vi "SwissSPAD Live_Get FLI Data Type for HDF5.vi"(8 "error in (no error)":errorcluster) -> (0 "error out":errorcluster, 3 "Data Type":string)   [LabVIEW 2021]
uses:
  SwissSPAD Live_Settings List.ctl
  SwissSPAD Live_SSx PCB Version.ctl
  SwissSPAD Live_SS2 DAQ Parameters 3.ctl
  SwissSPAD Live_SS2 Gate Definition.ctl
  SwissSPAD Live_SS3 DAQ Parameters.ctl
  SwissSPAD Live_SS3 Gate Definition.ctl
  SS3 Gate Width Definition Mode.ctl
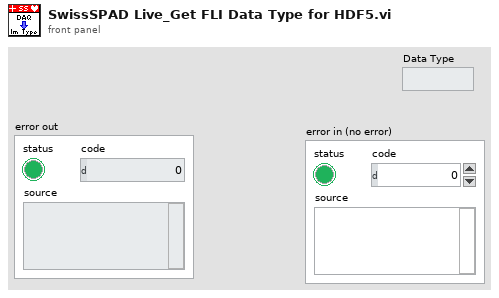
[diagram p1: front panel]
types:
  T1 = typedef "SwissSPAD Live_SSx PCB Version.ctl" = enum16{"unknown", "SS2 PCB1", "SS2 PCB2", "SS3 PCB1"}
  T2 = typedef "SwissSPAD Live_Settings List.ctl" = enum16{"FPGA:Bottom Half", "FPGA:Top Half", "FPGA:Bottom Bitfile Path", "FPGA:Top Bitfile Path", "FPGA:Bottom Bitstream Version", "FPGA:Top Bitstream Version", "FPGA:Auto Reset FPGA", "FPGA:Bottom FPGA Serial Number", "FPGA:Top FPGA Serial Number", "FPGA:Detector PCB Version", "Acquisition Parameters:Microlens", "Acquisition Parameters:SS2 DAQ Parameters", "Acquisition Parameters:Gate Configuration Array", "Acquisition Parameters:SS3 DAQ Parameters", "Acquisition Parameters:Buffer Size (# 8-bit Gates)", "File Information:File Information", "File Information:# Datasets in Series", "File Information:Scrambled File Flag", "File Information:SS3 Gate Slip Correction", "File Information:SS3 Hot Pixel Mismatch Detection", "File Information:Delay between Datasets", "File Information:Save Sum of All Gates Preview", "Image Parameters:Image ROI Information", "Image Parameters:Image Binning Options", "Image Parameters:SS3 Displayed Image", "Image Parameters:Image Display Options", "Image Parameters:Use Histogram Cursors", "Image Parameter:FPGA Data to Display", "UI Settings:Histogram Bins Number", "UI Settings:Histogram Bin Size", "UI Settings:Use Image Display Options", "UI Settings:Verbose Settings", "UI Settings:Verbose Saving"}
  T3 = typedef "SwissSPAD Live_SS2 DAQ Parameters 3.ctl" = cluster{"10 bits":bool, "# Exposure Sequences":u32, "# 1-bit Frame per Gate":u32, "Gate Shift":u32, "# Gates per Set":u32, "# Sets":u32, "Laser Period":dbl[unit], "Sync Period":dbl[unit], "Gate Offset":u32, "Auto-adjust Gate Offset":bool, "Gate Definition":T4, "Reversed Shift":bool}
  T4 = typedef "SwissSPAD Live_SS2 Gate Definition.ctl" = cluster{"gs_psincdec_0":u32, "gs_psincdec_1":u32, "gs_psincdec_2":u32, "gs_psincdec_3":u32, "gs_no_shift_adj_1":u32, "gs_no_shift_adj_2":u32, "gs_no_shift_adj_3":u32}
  T5 = typedef "SwissSPAD Live_SS3 DAQ Parameters.ctl" = cluster{"10 bits":bool, "# Exposure Sequences":u32, "# 1-bit Frame per Gate":u32, "Gate Shift":u32, "# Gate Pairs per Set":u32, "# Sets":u32, "Laser Period":dbl[unit], "Sync Period":dbl[unit], "Gate Offset":u32, "Auto-adjust Gate Offset":bool, "Gate Definition":T6, "Gate Width (ns)":dbl, "Reversed Shift":bool, "Intensity Mode":bool, "Gate Definition Mode":T7}
  T6 = typedef "SwissSPAD Live_SS3 Gate Definition.ctl" = cluster{"gs_psincdec_0":u32, "gs_psincdec_1":u32, "gs_no_shift_adj_1":u32, "gate_adj_2":u32}
  T7 = typedef "SS3 Gate Width Definition Mode.ctl" = enum32{"Item 0", "Item 1"}
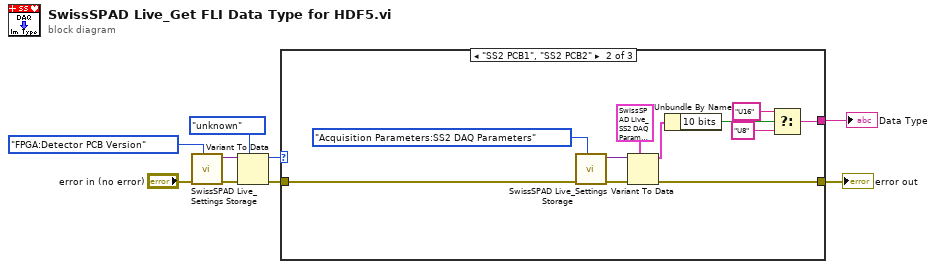
[diagram p0: block diagram]
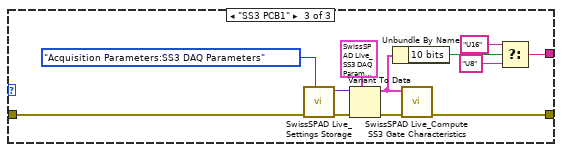
[diagram p3: hidden frame]
diagram:
  n1 = call "SwissSPAD Live_Settings Storage.vi"("Settings List"=SwissSPAD_Live_Settings_List."FPGA:Detector PCB Version", "Error In"="error in (no error)") -> ("Error Out"=w6:errorcluster, "Variant Data out"=w1:variant)  [unwired: 8 in]
  n2 = Variant To Data(error in=w6, type=SwissSPAD_Live_SSx_PCB_Version."unknown" ("Detector PCB Version"), Variant=w1) -> (data=w5:T1, error out=w4:errorcluster)
  n3 = case shown="\"SS2 PCB1\", \"SS2 PCB2\"" w5 {
    tunnel: [_ w21 w33] -> w9
    tunnel: w4 -> [w10 w13 w26]
    tunnel: [w10 w20 w24] -> w3
    frame "unknown", Default {
    }
    frame "SS2 PCB1", "SS2 PCB2" {
      n4 = call "SwissSPAD Live_Settings Storage.vi"("Settings List"=SwissSPAD_Live_Settings_List."Acquisition Parameters:SS2 DAQ Parameters", "Error In"=w13) -> ("Error Out"=w14:errorcluster, "Variant Data out"=w11:variant)  [unwired: 8 in]
      n5 = Variant To Data(error in=w14, type=T3 {"10 bits"=FALSE, "# Exposure Sequences"=0, "# 1-bit Frame per Gate"=0, "Gate Shift"=0, "# Gates per Set"=0, "# Sets"=1, "Laser Period"=0.0, "Sync Period"=0.0, "Gate Offset"=0, "Auto-adjust Gate Offset"=FALSE, "Gate Definition"={"gs_psincdec_0"=0, "gs_psincdec_1"=0, "gs_psincdec_2"=0, "gs_psincdec_3"=0, "gs_no_shift_adj_1"=0, "gs_no_shift_adj_2"=0, "gs_no_shift_adj_3"=0}, "Reversed Shift"=FALSE} ("SS2 DAQ Parameters"), Variant=w11) -> (data=w19:T3, error out=w20:errorcluster)
      n6 = Unbundle By Name(w19) -> ("10 bits"=w16:bool)
      n7 = Select(t="U16" ("name"), s=w16, f="U8" ("name")) -> (s? t:f=w21:string)
    }
    frame "SS3 PCB1" {
      n8 = call "SwissSPAD Live_Settings Storage.vi"("Settings List"=SwissSPAD_Live_Settings_List."Acquisition Parameters:SS3 DAQ Parameters", "Error In"=w26) -> ("Error Out"=w27:errorcluster, "Variant Data out"=w22:variant)  [unwired: 8 in]
      n9 = Variant To Data(error in=w27, type=T5 {"10 bits"=FALSE, "# Exposure Sequences"=0, "# 1-bit Frame per Gate"=0, "Gate Shift"=0, "# Gate Pairs per Set"=0, "# Sets"=1, "Laser Period"=0.0, "Sync Period"=0.0, "Gate Offset"=0, "Auto-adjust Gate Offset"=FALSE, "Gate Definition"={"gs_psincdec_0"=0, "gs_psincdec_1"=0, "gs_no_shift_adj_1"=0, "gate_adj_2"=0}, "Gate Width (ns)"=0.0, "Reversed Shift"=FALSE, "Intensity Mode"=FALSE, "Gate Definition Mode"=enum."Item 0"} ("SS3 DAQ Parameters"), Variant=w22) -> (data=w25:T5, error out=w32:errorcluster)
      n10 = Unbundle By Name(w25) -> ("10 bits"=w29:bool)
      n11 = call "SwissSPAD Live_Compute SS3 Gate Characteristics.vi"("Error In"=w32, "SS3 DAQ Parameters"=w25) -> ("Error Out"=w24:errorcluster)  [unwired: 8 in, 1 out]
      n12 = Select(t="U16" ("name"), s=w29, f="U8" ("name")) -> (s? t:f=w33:string)
    }
  }
  "Data Type" <- w9
  "error out" <- w3
